vi "Stop cRIO DAQ.vi"(5 "DAQ_AI_Reader endpoint":refnum<k21>, 7 "DAQ_CMD_Writer endpoint":refnum<k21>, 8 "error in (no error)":errorcluster) -> (0 "error out":errorcluster)   [LabVIEW 2024]
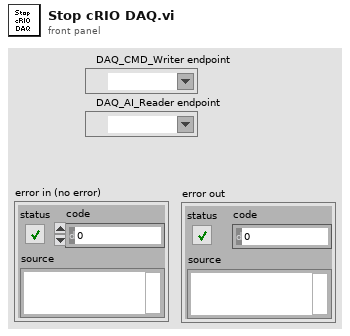
[diagram p1: front panel]
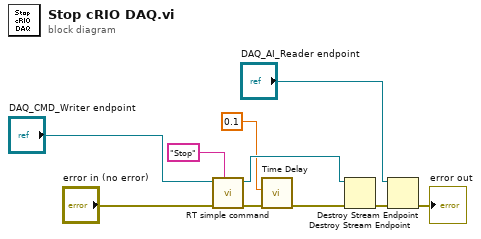
[diagram p0: block diagram]
diagram:
  n1 = call "RT simple command.vi"("Command"="Stop", "error in (no error)"="error in (no error)", "DAQ_CMD_Writer endpoint"="DAQ_CMD_Writer endpoint") -> ("error out"=w7:errorcluster, "DAQ_CMD_Writer endpoint out"=w3:refnum<k21>)  [unwired: 7 in]
  n2 = call "Time Delay"("error in (no error)"=w7, "Delay Time (s)"=0.1) -> ("error out"=w2:errorcluster)  [unwired: 9 in]
  n3 = Destroy Stream Endpoint(8:w2, 11:w3) -> (0:w9:errorcluster)
  n4 = Destroy Stream Endpoint(8:w9, 11:"DAQ_AI_Reader endpoint") -> (0:→"error out":errorcluster)
